vi "Shutdown.vi"(8 "error in":errorcluster, 11 "SwitchMatrix in":refnum<class "SwitchMatrix.lvclass">) -> (0 "error out":errorcluster, 3 "SwitchMatrix out":refnum<class "SwitchMatrix.lvclass">)   [LabVIEW 2019, in "SwitchMatrix.lvlib" / "SwitchMatrix.lvclass"]
doc: "This VI opens all switches in the matrix guaranteeing that there is no connection made when the device is reinilialized, and that it is being shut down with no connections made."
uses:
  Library/SwitchMatrix.lvclass
  builds/Instruments/Instruments.lvlibp/Library/Instruments.lvclass
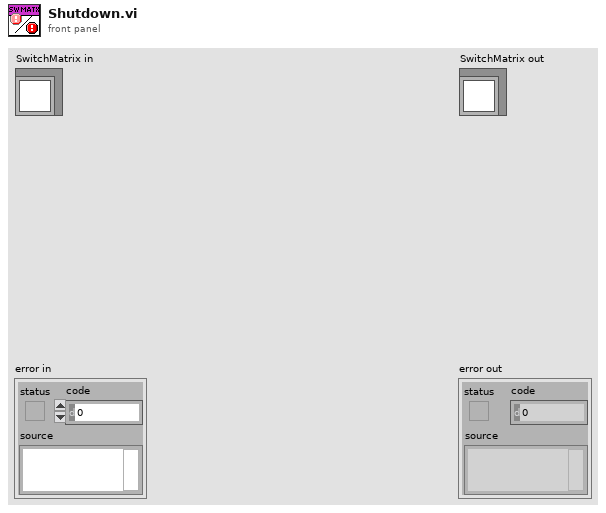
[diagram p1: front panel]
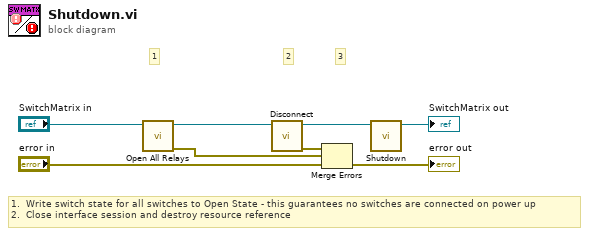
[diagram p0: block diagram]
diagram:
  # "1.  Write switch state for all switches to Open State - this guarantees no switches are connected on power up\n2.  Close interface session and destroy resource reference"
  # "3"
  # "2"
  # "1"
  n1 = call-dynamic "Open All Relays.vi"("SwitchMatrix in"="SwitchMatrix in") -> ("error out"=w4:errorcluster, "SwitchMatrix out"=w5:refnum<class "SwitchMatrix.lvclass">)  [unwired: 9 in]
  n2 = call-dynamic "Disconnect.vi"("SwitchMatrix in"=w5) -> ("error out"=w8:errorcluster, "SwitchMatrix out"=w2:refnum<class "SwitchMatrix.lvclass">)  [unwired: 9 in]
  n3 = Merge Errors(w8, w4, "error in") -> (→"error out":errorcluster)
  n4 = call-parent "Shutdown.vi"("Instruments in"=w2) -> ("Instruments out"=→"SwitchMatrix out":refnum<class "SwitchMatrix.lvclass">)  [unwired: 9 in, 1 out]
